vi "Get Subtype Description.vi"(8 "error in (no error)":errorcluster, 11 "Mouse Action in":refnum<class "Mouse Action.lvclass">) -> (0 "error out":errorcluster, 2 "Subtype Description":string, 3 "Mouse Action out":refnum<class "Mouse Action.lvclass">)   [LabVIEW 2020, in "MacroAssert.lvlib" / "Mouse Action.lvclass"]
uses:
  Mouse Action.lvclass
  Mouse Action.lvclass/Mouse Action.ctl
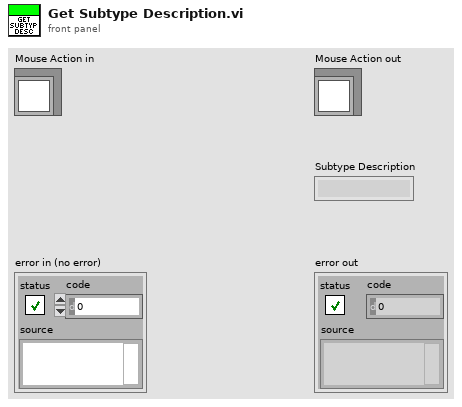
[diagram p1: front panel]
types:
  T1 = typedef "MacroAssert.lvlib/Mouse Action Type.ctl" = enum16{"Click", "Absolute Move", "Absolute Move and Click", "Relative Move", "Relative Move and Click", "Wheel Up", "Wheel Down"}
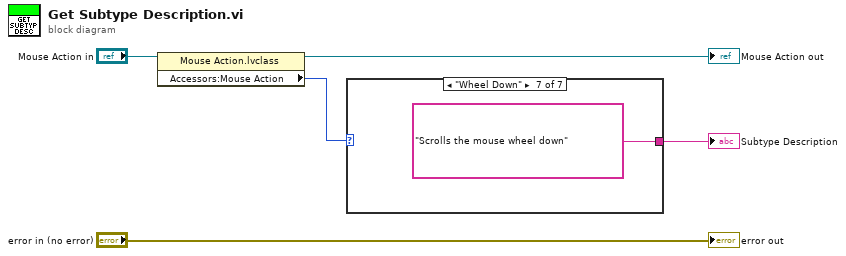
[diagram p0: block diagram]
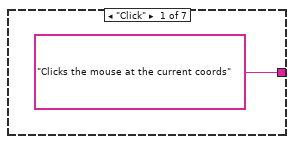
[diagram p2: hidden frame]
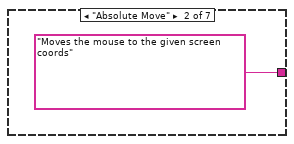
[diagram p3: hidden frame]
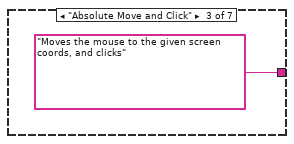
[diagram p4: hidden frame]
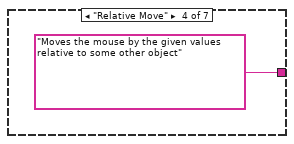
[diagram p5: hidden frame]
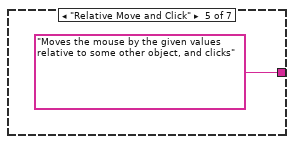
[diagram p6: hidden frame]
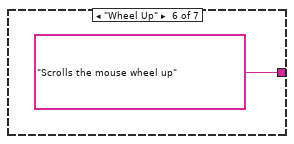
[diagram p7: hidden frame]
diagram:
  n1 = property class="Mouse Action.lvclass"(reference="Mouse Action in") -> (reference out=→"Mouse Action out":refnum<class "Mouse Action.lvclass">, "Accessors:Mouse Action"=w2:T1)  [unwired: 1 in, 1 out]
  n2 = case shown="\"Wheel Down\"" w2 {
    tunnel: ["Clicks the mouse at the current coords" "Moves the mouse to the given screen coords" "Moves the mouse to the given screen coords, and clicks" "Moves the mouse by the given values relative to some other object" "Moves the mouse by the given values relative to some other object, and clicks" "Scrolls the mouse wheel up" "Scrolls the mouse wheel down"] -> w1
    frame "Click" {
    }
    frame "Absolute Move" {
    }
    frame "Absolute Move and Click" {
    }
    frame "Relative Move" {
    }
    frame "Relative Move and Click" {
    }
    frame "Wheel Up" {
    }
    frame "Wheel Down" {
    }
  }
  "Subtype Description" <- w1
  "error out" <- "error in (no error)"
